vi "sudden change.vi"(0 "error in":dbl format="%#_13g", 1 "set point":dbl, 2 "speed min":bool, 3 "speed max":bool, 4 "no change":bool, 5 "sudden threshould":dbl=1.0 format="%#_13g") -> (16 "sudden change":bool)   [LabVIEW 2019]
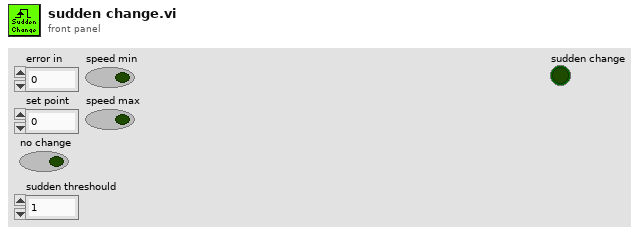
[diagram p1: front panel]
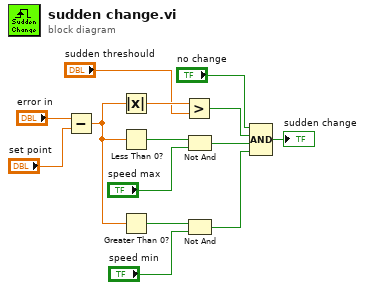
[diagram p0: block diagram]
diagram:
  n1 = Subtract(x="error in", y="set point") -> (x-y=w12:dbl)
  n2 = Absolute Value(x=w12) -> (abs(x)=w14:dbl)
  n3 = Less Than 0?(x=w12) -> (x < 0?=w11:bool)
  n4 = Greater Than 0?(x=w12) -> (x > 0?=w10:bool)
  n5 = Greater?(x=w14, y="sudden threshould") -> (0:w4:bool)
  n6 = Not And(1:"speed max", 2:w11) -> (0:w3:bool)
  n7 = Not And(1:"speed min", 2:w10) -> (0:w2:bool)
  n8 = Compound Arithmetic op=AND("no change", w4, w3, w2) -> (→"sudden change":bool)
